vi "init_parameters.vi"() -> (3 "String":string)   [LabVIEW 2018, in "ESP300.lvclass"]
uses:
  ESP300.lvclass
panel:
  in  "OK Button":bool
  in  "stage resource name":refnum<visa-resource-name>
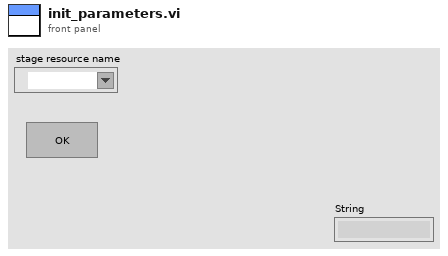
[diagram p1: front panel]
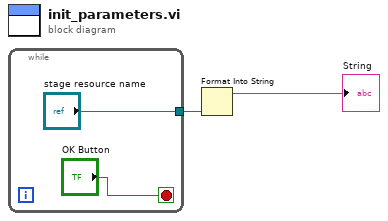
[diagram p0: block diagram]
diagram:
  n1 = while {
    tunnel: ["stage resource name"] -> w1
    stop <- "OK Button" stop-if-true
  }
  n2 = Format Into String(w1) -> (resulting string=→"String":string)  [unwired: 3 in, 1 out]
